vi "Revision Query.vi"(8 "error in (no error)":errorcluster, 11 "VISA Resource Name":refnum<visa-resource-name>) -> (0 "error out":errorcluster, 1 "Instr Firmware Revision":string, 2 "Instr Driver Revision":string, 3 "VISA Resource Name Out":refnum<visa-resource-name>)   [LabVIEW 2012, in "Agilent 34970.lvlib"]
doc: "This VI queries the current instrument firmware revision.\n\nRefer to hp34970a Readme.html for Instrument Driver Revision History and other Instrument Driver Information."
uses:
  <instrlib>/Agilent 34970/Agilent 34970.lvlib
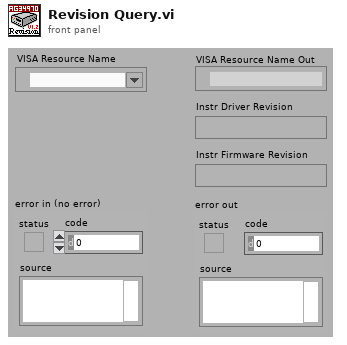
[diagram p1: front panel]
types:
  T1 = enum32{"invalid app kind", "Development System", "Run Time System", "Student Edition", "Embedded LabVIEW", "Evaluation", "Custom"}
  T2 = cluster{"Major":u16, "Minor":u16, "Fix":u16, "Build":u16}
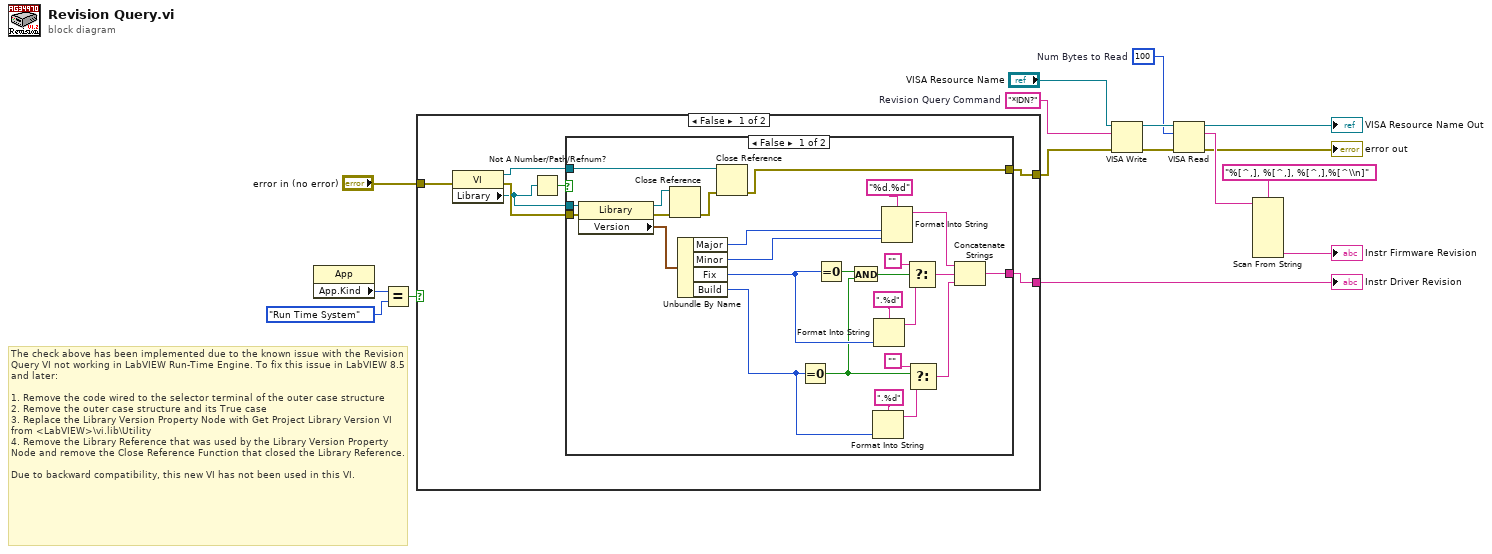
[diagram p0: block diagram]
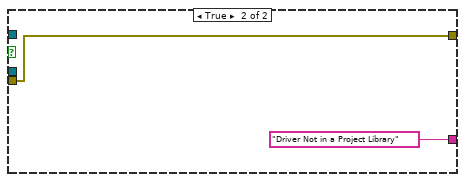
[diagram p2: hidden frame]
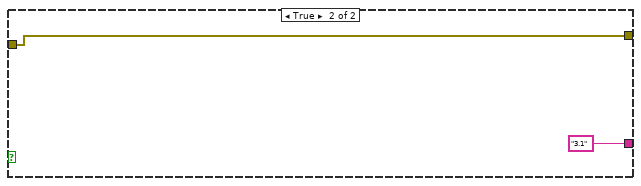
[diagram p3: hidden frame]
diagram:
  w1 = "*IDN?"  # Revision Query Command
  w11 = u32 100  # Num Bytes to Read
  # "The check above has been implemented due to the known issue with the Revision Query VI not working in LabVIEW Run-Time Engine. To fix this issue in LabVIEW 8.5 and later:\n\n1. Remove the code wired to the selector terminal of the outer case structure\n2. Remove the outer case structure and its True case\n3. Replace the Library Version Property Node with Get Project Library Version VI from <LabVIEW>\\vi.lib\\Utility\n4. Remove the Library Reference that was used by the Library Version Property Node and remove the Close Reference Function that closed the Library Reference.\n\nDue to backward compatibility, this new VI has not been used in this VI."
  n1 = property class="App"() -> ("App.Kind"=w3:T1)  [unwired: 2 in, 2 out]
  n2 = Equal?(x=w3, y=T1."Run Time System") -> (x = y?=w4:bool)
  n3 = case shown="False" w4 {
    tunnel: "error in (no error)" -> [w23 w53]
    tunnel: [w18 "3.1"] -> w6
    tunnel: [w17 w53] -> w5
    frame False {
      n4 = property class="VI"(error in=w23) -> (reference out=w19:refnum<vi>, error out=w22:errorcluster, "Library"=w21:refnum<vi>)  [unwired: 1 in]
      n5 = Not A Number/Path/Refnum?(number/path/refnum=w21) -> (NaN/Path/Refnum?=w20:bool)
      n6 = case shown="False" w20 {
        tunnel: [w28 w50] -> w17
        tunnel: [w27 "Driver Not in a Project Library"] -> w18
        tunnel: w22 -> [w26 w50]
        tunnel: w21 -> [w25 _]
        tunnel: w19 -> [w24 _]
        frame False {
          n7 = property class="Library"(reference=w25, error in=w26) -> (reference out=w48:refnum<vi>, error out=w49:errorcluster, "Version"=w46:T2)
          n8 = Close Reference(reference=w48, error in (no error)=w49) -> (error out=w47:errorcluster)
          n9 = Unbundle By Name(w46) -> ("Major"=w35:u16, "Minor"=w34:u16, "Fix"=w32:u16, "Build"=w33:u16)
          n10 = Close Reference(reference=w24, error in (no error)=w47) -> (error out=w28:errorcluster)
          n11 = Equal To 0?(x=w33) -> (x = 0?=w30:bool)
          n12 = Equal To 0?(x=w32) -> (x = 0?=w31:bool)
          n13 = And(x=w31, y=w30) -> (x .and. y?=w29:bool)
          n14 = Format Into String(format string=".%d", w33) -> (resulting string=w39:string)  [unwired: 2 in, 1 out]
          n15 = Format Into String(format string=".%d", w32) -> (resulting string=w43:string)  [unwired: 2 in, 1 out]
          n16 = Format Into String(format string="%d.%d", w35, w34) -> (resulting string=w41:string)  [unwired: 2 in, 1 out]
          n17 = Select(t="", s=w29, f=w43) -> (s? t:f=w40:string)
          n18 = Select(t="", s=w30, f=w39) -> (s? t:f=w36:string)
          n19 = Concatenate Strings(w41, w40, w36) -> (w27:string)
        }
        frame True {
        }
      }
    }
    frame True {
    }
  }
  "Instr Driver Revision" <- w6
  n20 = VISA Write(VISA resource name="VISA Resource Name", write buffer=w1, error in (no error)=w5) -> (VISA resource name out=w12:refnum<visa-resource-name>, error out=w13:errorcluster)  [unwired: 1 out]
  n21 = VISA Read(VISA resource name=w12, byte count=w11, error in (no error)=w13) -> (VISA resource name out=→"VISA Resource Name Out":refnum<visa-resource-name>, read buffer=w14:string, error out=→"error out":errorcluster)  [unwired: 1 out]
  n22 = Scan From String(format string="%[^,], %[^,], %[^,],%[^\\n]", input string=w14) -> (output 4=→"Instr Firmware Revision":string)  [unwired: 9 in, 3 out]
